vi "CRYMake Not Equal Name.vi"(8 "suffix IN":string, 9 "prefix In":string, 10 "Name In":string, 11 "Name array In":string[](array[string])) -> (3 "Name out":string)   [LabVIEW 2013]
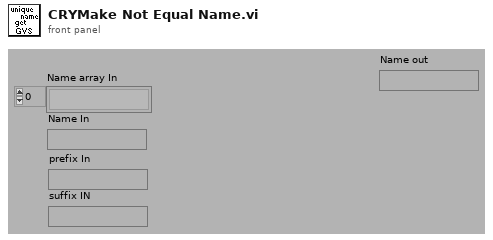
[diagram p1: front panel]
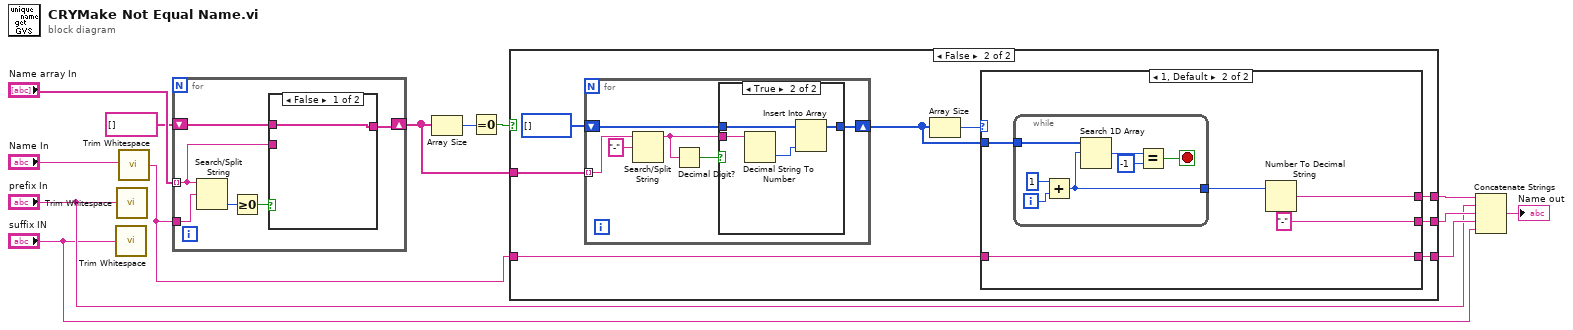
[diagram p0: block diagram]
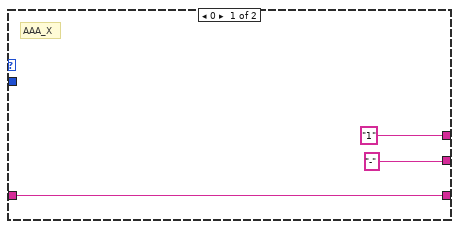
[diagram p4: hidden frame]
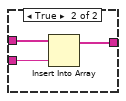
[diagram p5: hidden frame]
diagram:
  n1 = call <vilib>:"Trim Whitespace.vi"("string"="suffix IN") -> ()  [unwired: 1 in, 1 out]
  n2 = call <vilib>:"Trim Whitespace.vi"("string"="prefix In") -> ()  [unwired: 1 in, 1 out]
  n3 = call <vilib>:"Trim Whitespace.vi"("string"="Name In") -> ("trimmed string"=w9:string)  [unwired: 1 in]
  n4 = for {
    tunnel: "Name array In" -> [w14] mode=indexing
    tunnel: w9 -> [w19]
    shift-right: [w15] -> w7
    shift-left: string[] [] -> [w16]
    n5 = Search/Split String(string=w14, search string/char (-)=w19) -> (offset of match=w18:i32)  [unwired: 3 out]
    n6 = Greater Or Equal To 0?(x=w18) -> (x >= 0?=w17:bool)
    n7 = case shown="False" w17 {
      tunnel: w16 -> [w20 w23]
      tunnel: [w20 w22] -> w15
      tunnel: w14 -> [_ w21]
      frame False {
      }
      frame True {
        n8 = Insert Into Array(array=w23, new element=w21) -> (w22:string[])  [unwired: 1 in]
      }
    }
  }
  n9 = Array Size(array=w7) -> (size(s)=w11:i32)
  n10 = Equal To 0?(x=w11) -> (x = 0?=w10:bool)
  n11 = case shown="False" w10 {
    tunnel: w7 -> [_ w32]
    tunnel: w9 -> [w24 w29]
    tunnel: [_ w27] -> w6
    tunnel: [_ w26] -> w3
    tunnel: [w24 w25] -> w4
    frame True {
    }
    frame False {
      n12 = for {
        tunnel: w32 -> [w36] mode=indexing
        shift-right: [w37] -> w31
        shift-left: i32[] [] ("output array") -> [w38]
        n13 = Search/Split String(string=w36, search string/char (-)="-") -> (substring before match=w34:string)  [unwired: 3 out]
        n14 = Decimal Digit?(1:w34) -> (0:w33:bool)
        n15 = case shown="True" w33 {
          tunnel: w38 -> [w39 w42]
          tunnel: [w39 w41] -> w37
          tunnel: w34 -> [_ w43]
          frame False {
          }
          frame True {
            n16 = Decimal String To Number(string=w43) -> (number=w40:i32)  [unwired: 3 out]
            n17 = Insert Into Array(array=w42, new element=w40) -> (w41:i32[])  [unwired: 1 in]
          }
        }
      }
      n18 = Array Size(array=w31) -> (size(s)=w30:i32)
      n19 = case shown="1, Default" w30 {
        tunnel: w29 -> [w46 w48]
        tunnel: w31 -> [_ w51]
        tunnel: ["1" w50] -> w27
        tunnel: ["-" "-" ("string")] -> w26
        tunnel: [w46 w48] -> w25
        frame 0 {
          # "AAA_X"
        }
        frame 1, Default {
          n20 = while {
            tunnel: w51 -> [w58]
            tunnel: [w52] -> w47
            i -> [w54]
            stop <- w55 stop-if-true
            n21 = Add(x=1, y=w54) -> (x+y=w52:i32)
            n22 = Search 1D Array(1D array=w58, element=w52) -> (index of element=w57:i32)  [unwired: 1 out]
            n23 = Equal?(x=w57, y=-1) -> (x = y?=w55:bool)
          }
          n24 = Number To Decimal String(number=w47) -> (decimal integer string=w50:string)  [unwired: 1 out]
        }
      }
    }
  }
  n25 = Concatenate Strings(w6, "prefix In", w3, w4, "suffix IN") -> (→"Name out":string)
